vi "slopes2zern_test.vi"() -> ()   [LabVIEW 2018]
uses:
  <userlib>/WaveKit.lib/Controls/HasoSlopes.lvclass
panel:
  in  "idxType":enum16{"Wyant", "ANSI"}(ring)
  in  "Output folder":path=path "D:/Data/20200310"
  in  "Output file name":string="collar_p19_coeffs.txt"
  in  "Hasao slopes file":path=path "D:/Data/20200310/collar_p19.has"
  out "Zernike pupil":i32[][](graph)
  out "Measured pupil":i32[][](graph)
  out "Zernike Coefficients":dbl[](graph)
  out "error out":errorcluster
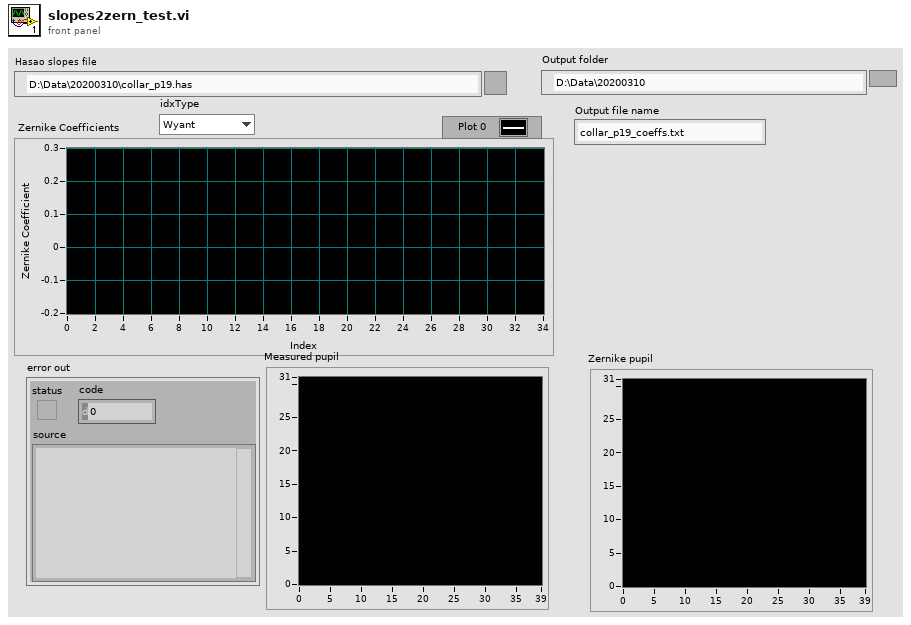
[diagram p1: front panel]
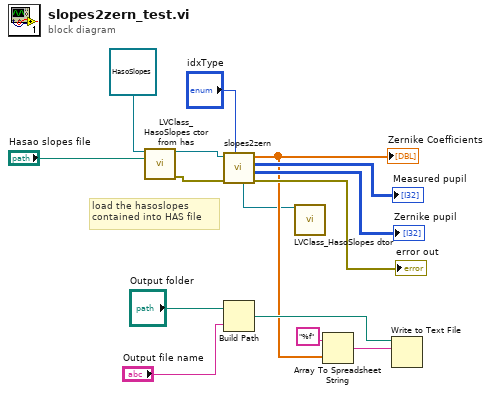
[diagram p0: block diagram]
diagram:
  # "load the hasoslopes\ncontained into HAS file"
  n1 = call <userlib>:"LVClass_HasoSlopes ctor from has.vi"("HasoSlopes in"=refnum<class "HasoSlopes.lvclass"> refnum, ".has path"="Hasao slopes file") -> ("HasoSlopes out"=w4:refnum<class "HasoSlopes.lvclass">, "error out"=w3:errorcluster)  [unwired: 12 in]
  n2 = call "slopes2zern.vi"("HasoSlopes in"=w4, "error in (no error)"=w3, "idxType"="idxType") -> ("HasoSlopes out"=w2:refnum<class "HasoSlopes.lvclass">, "Zernike Coefficients"=w7:dbl[], "Measured pupil"=→"Measured pupil":i32[][], "Zernike pupil"=→"Zernike pupil":i32[][], "error out"=→"error out":errorcluster)  [unwired: 3 in]
  "Zernike Coefficients" <- w7
  n3 = Build Path(base path="Output folder", name or relative path="Output file name") -> (appended path=w8:path)
  n4 = call <userlib>:"LVClass_HasoSlopes dtor.vi"("HasoSlopes in"=w2) -> ()  [unwired: 13 in, 2 out]
  n5 = Array To Spreadsheet String(array=w7, 3:"%f") -> (spreadsheet string=w11:string)  [unwired: 1 in]
  n6 = Write to Text File(file (use dialog)=w8, text=w11) -> ()  [unwired: 2 in, 3 out]
